vi "Set Field Units.vi"(1 "error in":T2, 2 "Field Units":u16(ring) items=["kG", "Tesla"], 3 "Communications Config":T1={"GPIB address"=22, "GPIB bus"=0, "connection ID"=refnum, "IP"="192.168.2.200", "Active Comm Interface"=0, "Serial Port"="", "Programmer Type"=0} {"Programmer Type" items=["Model 430", "Model 420"]; "Active Comm Interface" items=["TCP/IP (Model 430 Only)", "RS232", "IEEE488"]}) -> (0 "error out":T2)   [LabVIEW 2018]
panel:
  in  "GPIB Address":cluster{"GPIB address":i16, "GPIB bus":i16}={"GPIB address"=22, "GPIB bus"=0}
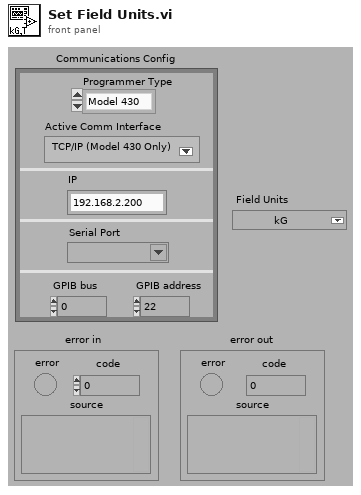
[diagram p1: front panel]
types:
  T1 = cluster{"GPIB address":i16, "GPIB bus":i16, "connection ID":refnum<k5>, "IP":string, "Active Comm Interface":u16, "Serial Port":refnum<visa-resource-name>, "Programmer Type":u16}
  T2 = cluster{"error":bool, "code":i32, "source":string}
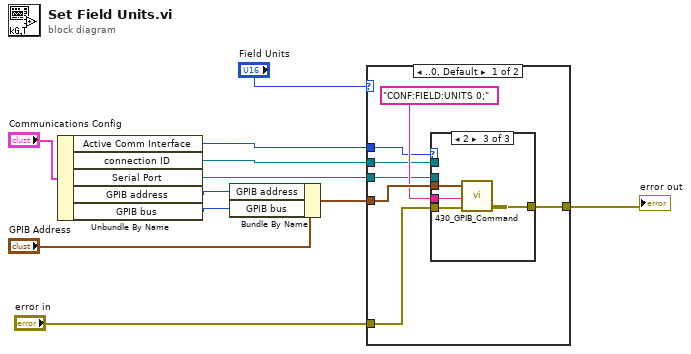
[diagram p0: block diagram]
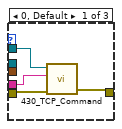
[diagram p2: hidden frame]
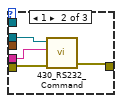
[diagram p3: hidden frame]
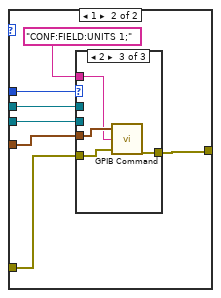
[diagram p4: hidden frame]
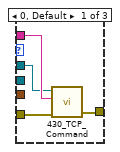
[diagram p5: hidden frame]
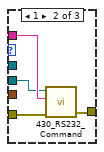
[diagram p6: hidden frame]
diagram:
  n1 = Unbundle By Name("Communications Config") -> ("Active Comm Interface"=w4:u16, "connection ID"=w3:refnum<k5>, "Serial Port"=w2:refnum<visa-resource-name>, "GPIB address"=w6:i16, "GPIB bus"=w5:i16)
  n2 = Bundle By Name(cluster="GPIB Address", "GPIB address"=w6, "GPIB bus"=w5) -> (w7:cluster{"GPIB address":i16, "GPIB bus":i16})
  n3 = case shown="..0, Default" "Field Units" {
    tunnel: w7 -> [w18 w37]
    tunnel: "error in" -> [w16 w35]
    tunnel: [w15 w34] -> w9
    tunnel: w4 -> [w14 w33]
    tunnel: w3 -> [w13 w32]
    tunnel: w2 -> [w12 w31]
    frame ..0, Default {
      n4 = case shown="2" w14 {
        tunnel: w18 -> [_ _ w30]
        tunnel: "CONF:FIELD:UNITS 0;" -> [w20 w24 w29]
        tunnel: w16 -> [w21 w25 w28]
        tunnel: [w22 w26 w27] -> w15
        tunnel: w13 -> [w19 _ _]
        tunnel: w12 -> [_ w23 _]
        frame 0, Default {
          n5 = call "430_TCP_Command.vi"("error in (no error)"=w21, "Command"=w20, "connection ID"=w19) -> ("error out"=w22:errorcluster)  [unwired: 1 in, 2 out]
        }
        frame 1 {
          n6 = call "430_RS232_Command.vi"("error in (no error)"=w25, "Command"=w24, "VISA resource name"=w23) -> ("error out"=w26:errorcluster)  [unwired: 1 in, 2 out]
        }
        frame 2 {
          n7 = call "430_GPIB_Command.vi"("GPIB (In)"=w30, "Input command"=w29, "error in"=w28) -> ("error out"=w27:T2)  [unwired: 3 out]
        }
      }
    }
    frame 1 {
      n8 = case shown="2" w33 {
        tunnel: w37 -> [_ _ w49]
        tunnel: "CONF:FIELD:UNITS 1;" -> [w39 w43 w48]
        tunnel: w35 -> [w40 w44 w47]
        tunnel: [w41 w45 w46] -> w34
        tunnel: w32 -> [w38 _ _]
        tunnel: w31 -> [_ w42 _]
        frame 0, Default {
          n9 = call "430_TCP_Command.vi"("error in (no error)"=w40, "Command"=w39, "connection ID"=w38) -> ("error out"=w41:errorcluster)  [unwired: 1 in, 2 out]
        }
        frame 1 {
          n10 = call "430_RS232_Command.vi"("error in (no error)"=w44, "Command"=w43, "VISA resource name"=w42) -> ("error out"=w45:errorcluster)  [unwired: 1 in, 2 out]
        }
        frame 2 {
          n11 = call "GPIB Command.vi"("GPIB (In)"=w49, "Input command"=w48, "error in"=w47) -> ("error out"=w46:T2)  [unwired: 3 out]
        }
      }
    }
  }
  "error out" <- w9
